vi "Wolna_Zapisz_Konf.vi"(8 "error in (no error)":errorcluster, 10 "Ustawienia do zapisu":T1[](array[typedef]), 11 "selected path":path) -> (0 "error out":errorcluster)   [LabVIEW 2014]
uses:
  Kontrolki/GUI/RejWol_konfig_opis GUI.ctl
  Kontrolki/GUI/RejWol_typ.ctl
  Kontrolki/GUI/RejWol_numer_kanalu.ctl
  <vilib>/Utility/config.llb/Write Key (String).vi
  <vilib>/Utility/config.llb/Write Key (U32).vi
  <vilib>/Utility/config.llb/NI_LVConfig.lvlib
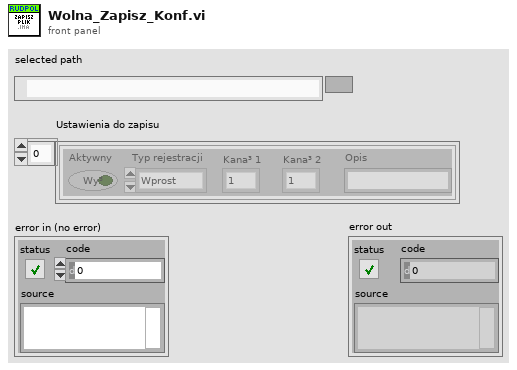
[diagram p1: front panel]
types:
  T1 = typedef "RejWol_konfig_opis GUI.ctl" = cluster{"Typ rejestracji":T2, "Opis":string, "Aktywny":bool, "Kana³ 1":T3, "Kana³ 2":T3}
  T2 = typedef "RejWol_typ.ctl" = enum16{"Wprost", "Modu³", "Kwadrat", "Iloczyn", "Faza"}
  T3 = typedef "RejWol_numer_kanalu.ctl" = enum16{"1", "2", "3", "4", "5", "6", "7", "8"}
  T4 = typedef "NI_LVConfig.lvlib/Config Data RefNum.ctl" = refnum<k1>
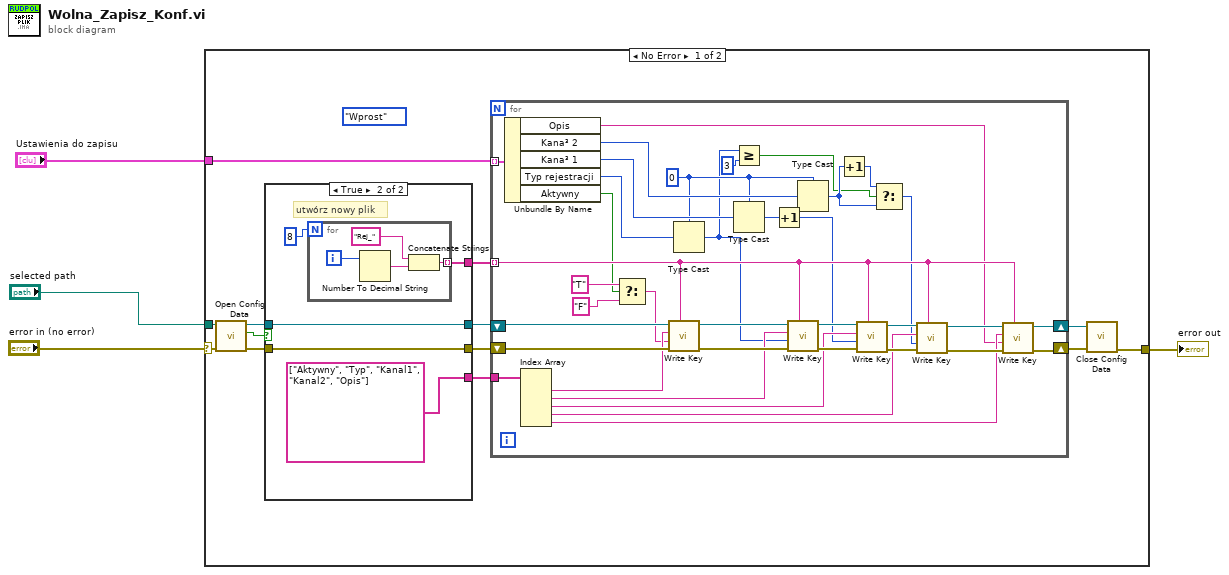
[diagram p0: block diagram]
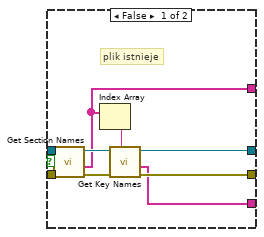
[diagram p2: hidden frame]
diagram:
  n1 = case shown="No Error" "error in (no error)" {
    selector: "error in (no error)" -> [w13 w73]
    tunnel: "Ustawienia do zapisu" -> [w17 _]
    tunnel: "selected path" -> [w14 _]
    tunnel: [w7 w73] -> w1
    frame No Error {
      (unwired) RejWol_typ."Wprost" ("Typ rejestracji")
      n2 = call <vilib>:"Open Config Data.vi"("error in (no error)"=w13, "configuration file path"=w14) -> ("error out"=w15:errorcluster, "file created?"=w5:bool, "refnum"=w16:T4)  [unwired: 7 in]
      n3 = case shown="True" w5 {
        tunnel: w16 -> [w26 w30]
        tunnel: w15 -> [w25 w31]
        tunnel: [w22 w31] -> w12
        tunnel: [w21 w30] -> w11
        tunnel: [w20 w27] -> w10
        tunnel: [w18 string[] ["Aktywny", "Typ", "Kanal1", "Kanal2", "Opis"] ("key names 2")] -> w6
        frame False {
          # "plik istnieje"
          n4 = call <vilib>:"Get Section Names.vi"("error in (no error)"=w25, "refnum"=w26) -> ("error out"=w23:errorcluster, "section names"=w20:string[], "refnum out"=w24:T4)  [unwired: 7 in]
          n5 = Index Array(array=w20) -> (element=w19:string)  [unwired: 1 in]
          n6 = call <vilib>:"Get Key Names.vi"("section"=w19, "error in (no error)"=w23, "refnum"=w24) -> ("error out"=w22:errorcluster, "key names"=w18:string[], "refnum out"=w21:T4)  [unwired: 5 in, 1 out]
        }
        frame True {
          # "utwórz nowy plik"
          n7 = for {
            N: 8 -> [_]
            tunnel: [w34] -> w27 mode=indexing
            i -> [w35]
            n8 = Number To Decimal String(number=w35) -> (decimal integer string=w33:string)  [unwired: 1 in]
            n9 = Concatenate Strings("Rej_", w33) -> (w34:string)
          }
        }
      }
      n10 = for {
        tunnel: w10 -> [w53] mode=indexing
        tunnel: w17 -> [w72] mode=indexing
        tunnel: w6 -> [w59]
        shift-right: [w66] -> w8
        shift-left: w11 -> [w71]
        shift-right: [w65] -> w9
        shift-left: w12 -> [w64]
        w44 = u16 0
        n11 = Unbundle By Name(w72) -> ("Opis"=w49:string, "Kana³ 2"=w45:T3, "Kana³ 1"=w46:T3, "Typ rejestracji"=w47:T2, "Aktywny"=w48:bool)
        n12 = Index Array(array=w59) -> (element #1=w58:string, element #2=w57:string, element #3=w56:string, element #4=w55:string, element #5=w54:string)  [unwired: 5 in]
        n13 = Select(t="T", s=w48, f="F") -> (s? t:f=w52:string)
        n14 = call-poly <vilib>:"Write Key.vi"("section"=w53, "error in (no error)"=w64, "value"=w52, "key"=w58, "refnum"=w71) -> ("error out"=w63:errorcluster, "refnum out"=w70:T4)  [unwired: 4 in, 1 out]
        n15 = Type Cast(type=w44, x=w47) -> (*(type *) &x=w37:u16)
        n16 = Greater Or Equal?(x=w37, y=u16 3) -> (x >= y?=w38:bool)
        n17 = Type Cast(type=w44, x=w46) -> (*(type *) &x=w43:u16)
        n18 = Increment(x=w43) -> (x+1=w42:u16)
        n19 = call-poly <vilib>:"Write Key.vi"("section"=w53, "error in (no error)"=w63, "value"=w37, "key"=w57, "refnum"=w70) -> ("error out"=w62:errorcluster, "refnum out"=w69:T4)  [unwired: 4 in, 1 out]
        n20 = Type Cast(type=w44, x=w45) -> (*(type *) &x=w39:u16)
        n21 = Increment(x=w39) -> (x+1=w40:u16)
        n22 = call-poly <vilib>:"Write Key.vi"("section"=w53, "error in (no error)"=w62, "value"=w42, "key"=w56, "refnum"=w69) -> ("error out"=w61:errorcluster, "refnum out"=w68:T4)  [unwired: 4 in, 1 out]
        n23 = Select(t=w40, s=w38, f=w39) -> (s? t:f=w41:u16)
        n24 = call-poly <vilib>:"Write Key.vi"("section"=w53, "error in (no error)"=w61, "value"=w41, "key"=w55, "refnum"=w68) -> ("error out"=w60:errorcluster, "refnum out"=w67:T4)  [unwired: 4 in, 1 out]
        n25 = call-poly <vilib>:"Write Key.vi"("section"=w53, "error in (no error)"=w60, "value"=w49, "key"=w54, "refnum"=w67) -> ("error out"=w65:errorcluster, "refnum out"=w66:T4)  [unwired: 4 in, 1 out]
      }
      n26 = call <vilib>:"Close Config Data.vi"("error in (no error)"=w9, "refnum"=w8) -> ("error out"=w7:errorcluster)  [unwired: 8 in, 1 out]
    }
    frame Error {
    }
  }
  "error out" <- w1
